vi "Kinimatics_Update Pose from Twist.vi"(9 "TWIST":T1, 11 "POSE":T2 {"ROTATION"."SIN" format="%13.4f"; "ROTATION"."COS" format="%13.4f"; "ROTATION"."VALUE" format="%13.4f"; "TRANSLATION"."Y" format="%14.3f"; "TRANSLATION"."X" format="%14.3f"}) -> (3 "UpdatedPose":T2 {"ROTATION"."SIN" format="%13.4f"; "ROTATION"."COS" format="%13.4f"; "ROTATION"."VALUE" format="%13.4f"; "TRANSLATION"."Y" format="%14.3f"; "TRANSLATION"."X" format="%14.3f"})   [LabVIEW 2020, in "Swerve_Odometry_SEN.lvlib"]
doc: "Obtain a new Pose2d from a (constant curvature) velocity.\n\nSee <a href=\"https://file.tavsys.net/control/state-space-guide.pdf\"> Controls Engineering in the FIRST Robotics Competition</a> section on nonlinear pose estimation for derivation.\n\nThe twist is a change in pose in the robot's coordinate frame since the previous pose update. When the user runs exp() on the previous known field-relative pose with the argument being the twist, the user will receive the new field-relative pose.\n\n\"Exp\" represents the pose exponential, which is solving a differential equation moving the pose forward in time.\n\nPARAMETERS:\n--------------\n - POSE - current POSE data structure\n - TWIST - The change in pose in the robot's coordinate frame since the previous pose update. For example, if a non-holonomic robot moves forward 0.01 meters and changes angle by 0.5 degrees since the previous pose update, the twist would be Twist2d{0.01, 0.0, toRadians(0.5)}\n\nRETURNS:\n-----------\n- OUT POSE - The new pose of the robot."
uses:
  Swerve_Odometry_SEN.lvlib
  Cluster_TRANSLATION2D.ctl
  Cluster_ROTATION2D.ctl
  Cluster_TRANSFORM2D.ctl
  Cluster_POSE2D.ctl
  Cluster_TWIST2D.ctl
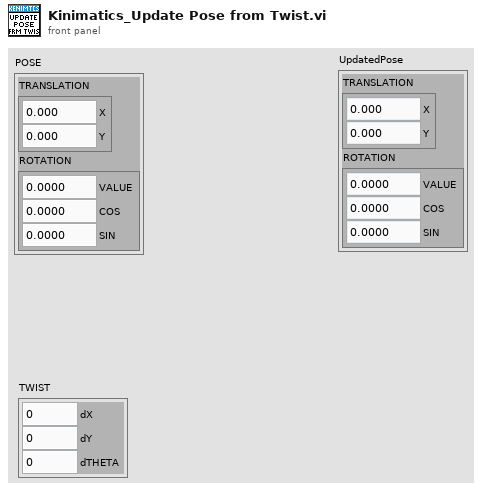
[diagram p1: front panel]
types:
  T1 = typedef "Swerve_Odometry_SEN.lvlib/Cluster_TWIST2D.ctl" = cluster{"dX":dbl, "dY":dbl, "dTHETA":dbl}
  T2 = typedef "Swerve_Odometry_SEN.lvlib/Cluster_POSE2D.ctl" = cluster{"TRANSLATION":T3, "ROTATION":T4}
  T3 = typedef "Swerve_Odometry_SEN.lvlib/Cluster_TRANSLATION2D.ctl" = cluster{"X":dbl, "Y":dbl}
  T4 = typedef "Swerve_Odometry_SEN.lvlib/Cluster_ROTATION2D.ctl" = cluster{"VALUE":dbl, "COS":dbl, "SIN":dbl}
  T5 = typedef "Swerve_Odometry_SEN.lvlib/Cluster_TRANSFORM2D.ctl" = cluster{"TRANSLATION":T3, "ROTATION":T4, "xF":bool}
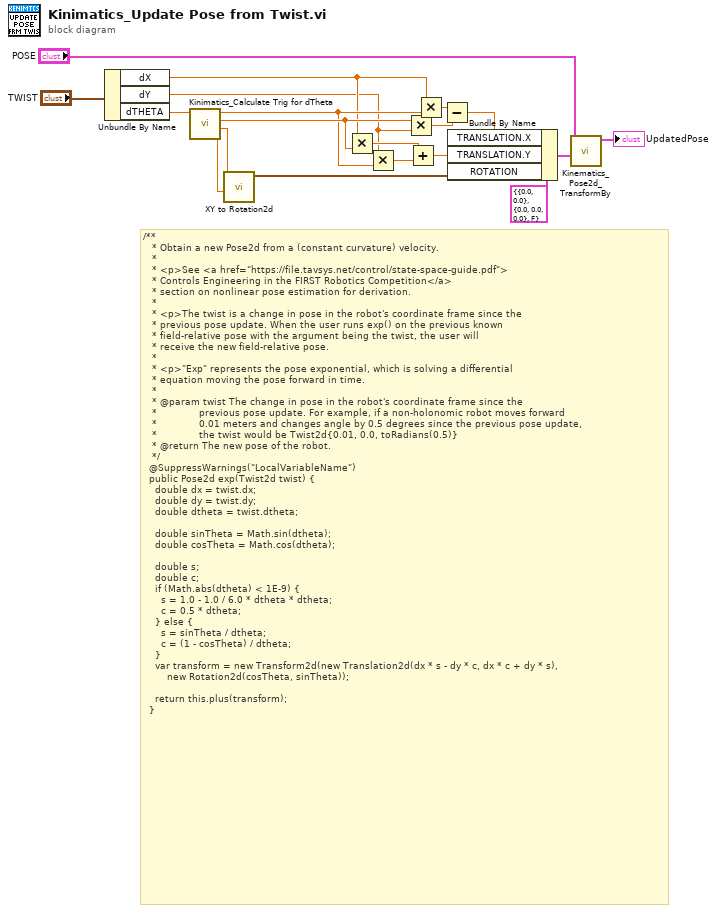
[diagram p0: block diagram]
diagram:
  # "/**\n   * Obtain a new Pose2d from a (constant curvature) velocity.\n   *\n   * <p>See <a href=\"https://file.tavsys.net/control/state-space-guide.pdf\">\n   * Controls Engineering in the FIRST Robotics Competition</a>\n   * section on nonlinear pose estimation for derivation.\n   *\n   * <p>The twist is a change in pose in the robot's coordinate frame since the\n   * previous pose update. When the user runs exp() on the previous known\n   * field-relative pose with the argument being the twist, the user will\n   * receive the new field-relative pose.\n   *\n   * <p>\"Exp\" represents the pose exponential, which is solving a differential\n   * equation moving the pose forward in time.\n   *\n   * @param twist The change in pose in the robot's coordinate frame since the\n   *              previous pose update. For example, if a non-holonomic robot moves forward\n   *              0.01 meters and changes angle by 0.5 degrees since the previous pose update,\n   *              the twist would be Twist2d{0.01, 0.0, toRadians(0.5)}\n   * @return The new pose of the robot.\n   */\n  @SuppressWarnings(\"LocalVariableName\")\n  public Pose2d exp(Twist2d twist) {\n    double dx = twist.dx;\n    double dy = twist.dy;\n    double dtheta = twist.dtheta;\n\n    double sinTheta = Math.sin(dtheta);\n    double cosTheta = Math.cos(dtheta);\n\n    double s;\n    double c;\n    if (Math.abs(dtheta) < 1E-9) {\n      s = 1.0 - 1.0 / 6.0 * dtheta * dtheta;\n      c = 0.5 * dtheta;\n    } else {\n      s = sinTheta / dtheta;\n      c = (1 - cosTheta) / dtheta;\n    }\n    var transform = new Transform2d(new Translation2d(dx * s - dy * c, dx * c + dy * s),\n        new Rotation2d(cosTheta, sinTheta));\n\n    return this.plus(transform);\n  }"
  n1 = Unbundle By Name("TWIST") -> ("dX"=w11:dbl, "dY"=w10:dbl, "dTHETA"=w9:dbl)
  n2 = call "Kinimatics_Calculate Trig for dTheta.vi"("DTHETA"=w9) -> ("Cos Of DTheta Out"=w1:dbl, "Sin Of DTheta Out"=w13:dbl, "Cosine/dTheta Out"=w19:dbl, "Sin/dTheta Out"=w16:dbl)  [unwired: 7 in]
  n3 = call "XY to Rotation2d.vi"("Y or sine"=w1, "X or  cosine"=w13) -> ("ROTATION"=w7:T4)  [unwired: 9 in]
  n4 = Multiply(x=w11, y=w19) -> (x*y=w15:dbl)
  n5 = Multiply(x=w10, y=w16) -> (x*y=w14:dbl)
  n6 = Multiply(x=w19, y=w10) -> (x*y=w17:dbl)
  n7 = Add(x=w15, y=w14) -> (x+y=w3:dbl)
  n8 = Multiply(x=w11, y=w16) -> (x*y=w18:dbl)
  n9 = Subtract(x=w18, y=w17) -> (x-y=w2:dbl)
  n10 = Bundle By Name(cluster=T5 {"TRANSLATION"={"X"=0.0, "Y"=0.0}, "ROTATION"={"VALUE"=0.0, "COS"=0.0, "SIN"=0.0}, "xF"=FALSE} ("TRANSFORM"), "TRANSLATION.X"=w2, "TRANSLATION.Y"=w3, "ROTATION"=w7) -> (w5:T5)
  n11 = call "Kinematics_Pose2d_TransformBy.vi"("Other TRANSFORM"=w5, "In POSE"="POSE") -> ("Out POSE Out"=→"UpdatedPose":T2)  [unwired: 9 in]
